vi "SECoP_dataGetAdditionalInteger.vi"(7 "Position":u32, 8 "error in (no error)":errorcluster, 9 "Index":u32, 10 "SECoP_dataPtr":T1 {"ptr64" format="%.0x"; "ptr32" format="%.0x"}, 11 "DLL path (in)":T2) -> (0 "error out":errorcluster, 2 "Value":i64, 3 "DLL path (out)":T2)   [LabVIEW 2023, in "SECoP.lvlib"]
doc: "Call <b>\"SECoP_dataGetAdditionalInteger.vi\"</b> to retrieve the numeric value (integer) of an additional item of SECoP_dataPtr, selected by index.\n\n<b>DLL path</b> input and output of cluster from \"SECoP-Initialize.vi\"\n<b>SECoP_dataPtr</b> data to access\n<b>Position</b> points to a virtual flattened entry of the data type\n<b>Index</b> zero based index to additional item of SECoP_dataPtr\n<b>Value</b> numeric value"
uses:
  SECoP.lvlib
  SECoP-libraries.ctl
  SECoP-data.ctl
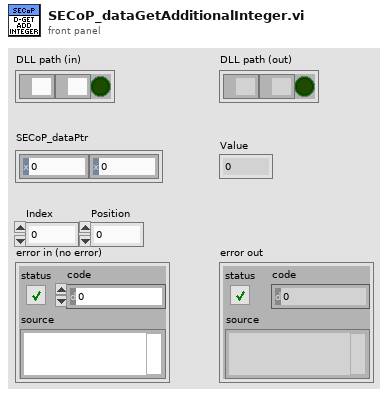
[diagram p1: front panel]
types:
  T1 = typedef "SECoP.lvlib/SECoP-data.ctl" = cluster{"ptr32":u32, "ptr64":u64}
  T2 = typedef "SECoP.lvlib/SECoP-libraries.ctl" = cluster{"serverDLL":path, "variantDLL":path, "cleanup_mode":bool}
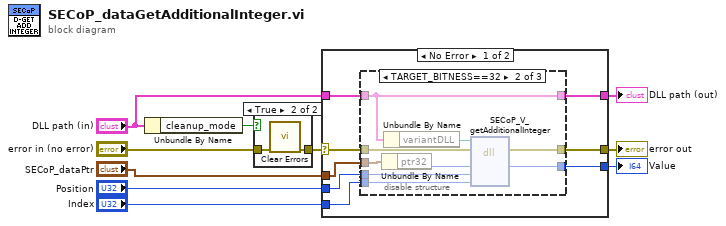
[diagram p0: block diagram]
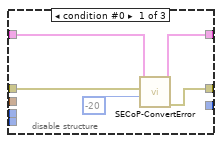
[diagram p3: hidden frame]
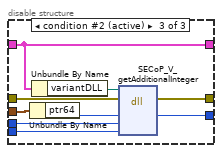
[diagram p4: hidden frame]
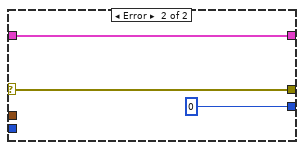
[diagram p5: hidden frame]
diagram:
  n1 = Unbundle By Name("DLL path (in)") -> ("cleanup_mode"=w7:bool)
  n2 = case shown="True" w7 {
    tunnel: "error in (no error)" -> [w11 w13]
    tunnel: [w11 w12] -> w5
    frame False {
    }
    frame True {
      n3 = call <vilib>:"Clear Errors.vi"("error in (no error)"=w13) -> ("error out"=w12:errorcluster)  [unwired: 5 in, 1 out]
    }
  }
  n4 = case shown="No Error" w5 {
    selector: w5 -> [w21 w46]
    tunnel: "DLL path (in)" -> [w20 w47]
    tunnel: [w15 w47] -> w9
    tunnel: [w14 w46] -> w8
    tunnel: "Position" -> [w19 _]
    tunnel: "Index" -> [w18 _]
    tunnel: [w17 i64 0 ("Value")] -> w2
    tunnel: "SECoP_dataPtr" -> [w16 _]
    frame No Error {
      n5 = disable-structure shown="TARGET_BITNESS==32" {
        disable-tunnel: w21 -> [w24 w35 w44]
        disable-tunnel: w20 -> [w26 w27 w36]
        disable-tunnel: [w25 w27 w36] -> w15
        disable-tunnel: [w22 w34 w43] -> w14
        disable-tunnel: w19 -> [_ w33 w42]
        disable-tunnel: w18 -> [_ w32 w41]
        disable-tunnel: [_ w29 w38] -> w17
        disable-tunnel: w16 -> [_ w30 w39]
        frame condition #0 {
          n6 = call "SECoP-ConvertError.vi"("return code"=-20, "error in (no error)"=w24, "DLL path (in)"=w26) -> ("error out"=w22:errorcluster, "DLL path (out)"=w25:T2)  [unwired: 7 in]
        }
        frame condition #1 {
          n7 = Unbundle By Name(w30) -> ("ptr32"=w31:u32)
          n8 = Unbundle By Name(w27) -> ("variantDLL"=w28:path)
          n9 = dll-call lib="Z:/Praktische_Aufgaben/SECoP-LabVIEW2015/32bit/SECoP32.dll" fn="SECoP_V_getAdditionalInteger"(path in=w28, error in=w35, "pData"=w31, "uPosition"=w33, "uIndex"=w32) -> (error out=w34:errorcluster, "return type"=w29:i64)  [unwired: 4 in, 1 out]
        }
        frame condition #2 (active) {
          n10 = Unbundle By Name(w39) -> ("ptr64"=w40:u64)
          n11 = Unbundle By Name(w36) -> ("variantDLL"=w37:path)
          n12 = dll-call lib="Z:/Praktische_Aufgaben/SECoP-LabVIEW2015/32bit/SECoP32.dll" fn="SECoP_V_getAdditionalInteger"(path in=w37, error in=w44, "pData"=w40, "uPosition"=w42, "uIndex"=w41) -> (error out=w43:errorcluster, "return type"=w38:i64)  [unwired: 4 in, 1 out]
        }
      }
    }
    frame Error {
    }
  }
  "DLL path (out)" <- w9
  "error out" <- w8
  "Value" <- w2
